vi "Save angle file.vi"(8 "error in (no error)":errorcluster, 10 "prompt":string, 11 "Angle chart":cluster{"Angle":dbl, "Data":dbl}[](array[cluster])) -> (0 "error out":errorcluster)   [LabVIEW 2020]
uses:
  <vilib>/Utility/sysdir.llb/System Directory Type.ctl
panel:
  out "String":string
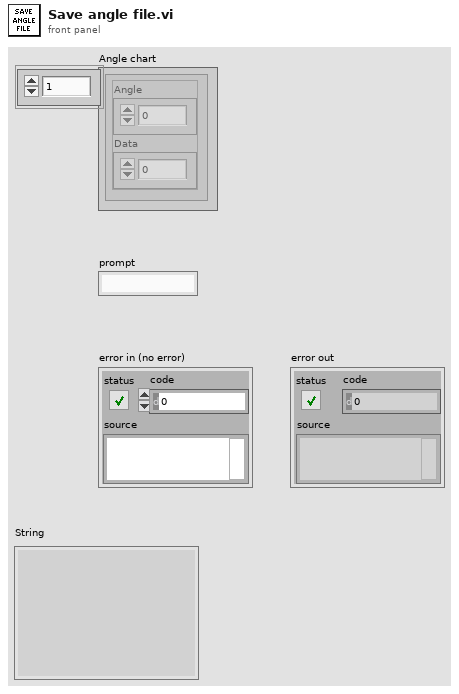
[diagram p1: front panel]
types:
  T1 = enum16{"open", "replace", "create", "open or create", "replace or create", "replace or create with confirmation"}
  T2 = typedef "System Directory Type.ctl" = i32
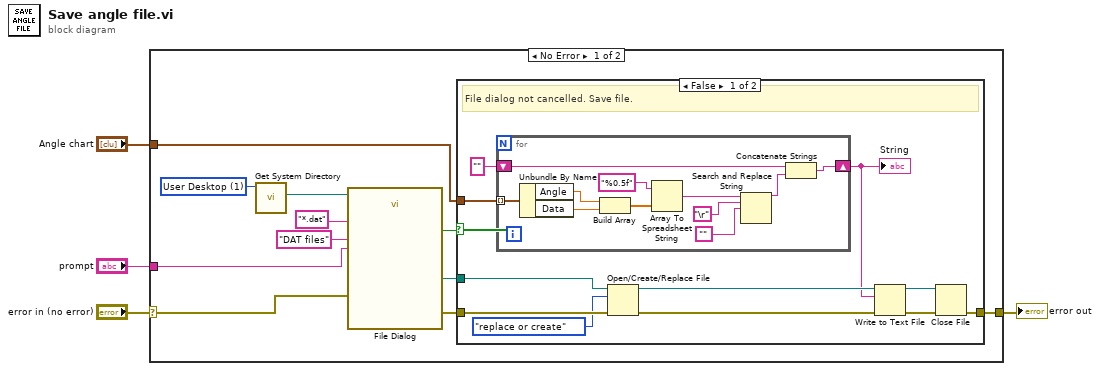
[diagram p0: block diagram]
diagram:
  n1 = case shown="No Error" "error in (no error)" {
    selector: "error in (no error)" -> [w15 w39]
    tunnel: [w9 w39] -> w3
    tunnel: "Angle chart" -> [w8 _]
    tunnel: "prompt" -> [w5 _]
    frame No Error {
      w14 = T2 1 items=["User Home"=0, "User Desktop"=1, "User Documents"=2, "User Application Data"=3, "User Preferences"=4, "User Temporary"=5, "Public Documents"=6, "Public Application Data"=7, "Public Preferences"=8, "Public Cache"=13, "System Core Libraries"=9, "System Installed Libraries"=10, "Application Files"=11, "Boot Volume Root"=12] ("system directory type")
      n2 = call <vilib>:"Get System Directory.vi"("system directory type"=w14) -> ("system directory"=w13:path)  [unwired: 10 in]
      n3 = call "File Dialog"("start path"=w13, "prompt"=w5, "error in"=w15, "pattern (all files)"="*.dat" ("pattern label"), "pattern label"="DAT files") -> ("selected path"=w7:path, "cancelled"=w10:bool, "error out"=w11:errorcluster)  [unwired: 7 in, 1 out]
      n4 = case shown="False" w10 {
        tunnel: w11 -> [w24 w38]
        tunnel: [w18 w38] -> w9
        tunnel: w8 -> [w26 _]
        tunnel: w7 -> [w23 _]
        frame False {
          # "File dialog not cancelled. Save file."
          n5 = for {
            tunnel: w26 -> [w37] mode=indexing
            shift-right: [w31] -> w19
            shift-left: "" -> [w32]
            n6 = Unbundle By Name(w37) -> ("Angle"=w35:dbl, "Data"=w34:dbl)
            n7 = Build Array(w35, w34) -> (w33:dbl[])
            n8 = Array To Spreadsheet String(array=w33, 3:"%0.5f" ("format string")) -> (spreadsheet string=w30:string)  [unwired: 1 in]
            n9 = Search and Replace String(input string=w30, search string="\r", replace string="") -> (result string=w29:string)  [unwired: 5 in, 3 out]
            n10 = Concatenate Strings(w32, w29) -> (w31:string)
          }
          "String" <- w19
          n11 = Open/Create/Replace File(file path (use dialog)=w23, error in=w24, operation (0:open)=T1."replace or create") -> (refnum out=w20:refnum<file>, error out=w22:errorcluster)  [unwired: 3 in, 1 out]
          n12 = Write to Text File(file (use dialog)=w20, text=w19, error in=w22) -> (refnum out=w17:refnum<file>, error out=w21:errorcluster)  [unwired: 1 in, 1 out]
          n13 = Close File(refnum=w17, error in=w21) -> (error out=w18:errorcluster)  [unwired: 1 out]
        }
        frame True {
          # "Dialog cancelled. Do nothing."
        }
      }
    }
    frame Error {
    }
  }
  "error out" <- w3
